vi "numeros de 0 a 1.vi"() -> ()   [LabVIEW 2020]
panel:
  in  "Numeric 2":i32
  out "I":dbl
  out "Numbers (0 a 1 )":dbl
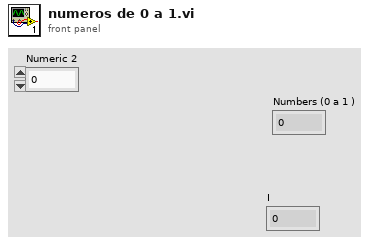
[diagram p1: front panel]
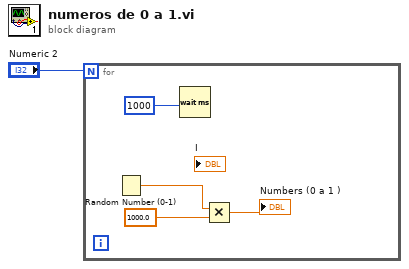
[diagram p0: block diagram]
diagram:
  n1 = for {
    N: "Numeric 2" -> [_]
    n2 = Random Number (0-1)() -> (number: 0 to 1=w3:dbl)
    n3 = Wait (ms)(milliseconds to wait=1000) -> ()  [unwired: 1 out]
    n4 = Multiply(x=w3, y=1000.0) -> (x*y=→"Numbers (0 a 1 )":dbl)
  }
